vi "Set Relative Sizes.vi"(8 "error in (no error)":errorcluster, 10 "Relative sizes":dbl[](array[numeric]), 11 "Divider in":refnum<class "Divider.lvclass">) -> (0 "error out":errorcluster, 3 "Divider out":refnum<class "Divider.lvclass">)   [LabVIEW 2021, in "Divider.lvclass"]
doc: "Copyright 2018, Wiebe Walstra, wiebe@carya.nl."
uses:
  Divider.lvclass
  Divider.lvclass/Divider.ctl
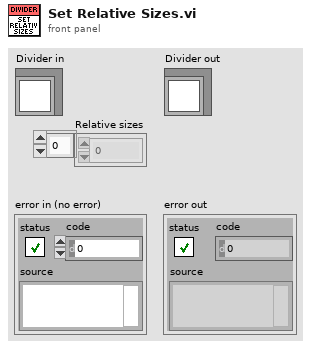
[diagram p1: front panel]
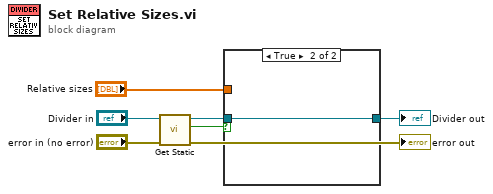
[diagram p0: block diagram]
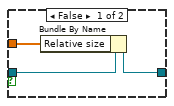
[diagram p2: hidden frame]
diagram:
  n1 = call-dynamic "Get Static.vi"("error in (no error)"="error in (no error)", "Divider in"="Divider in") -> ("error out"=→"error out":errorcluster, "Static?"=w1:bool, "Divider out"=w2:refnum<class "Divider.lvclass">)  [unwired: 7 in]
  n2 = case shown="True" w1 {
    tunnel: [w10 w11] -> w6
    tunnel: "Relative sizes" -> [w9 _]
    tunnel: w2 -> [w8 w11]
    frame False {
      n3 = Bundle By Name(cluster=w8, "Relative size"=w9) -> (w10:refnum<class "Divider.lvclass">)
    }
    frame True {
    }
  }
  "Divider out" <- w6
